vi "Event-Driven State Machine - Handle Error Locally.vi"() -> ()   [LabVIEW 2020]
uses:
  support/States.ctl
  support/State Machine Data.ctl
  <vilib>/DAQmx/read.llb/DAQmx Read (Analog 2D DBL NChan NSamp).vi
  <vilib>/DAQmx/write.llb/DAQmx Write (Analog DBL 1Chan 1Samp).vi
  <vilib>/DAQmx/create/channels.llb/DAQmx Create Channel (AI-Voltage-Basic).vi
  <vilib>/DAQmx/configure/timing.llb/DAQmx Timing (Sample Clock).vi
  <vilib>/DAQmx/miscellaneous.llb/DAQmx Fill In Error Info.vi
  <vilib>/Utility/file.llb/Write Delimited Spreadsheet (DBL).vi
  <vilib>/DAQmx/create/channels.llb/DAQmx Create Channel (AO-Voltage-Basic).vi
panel:
  in  "AO Voltage Channel":tag="PCI-6221/ao1"
  in  "Generate Stimulus":bool
  out "Threshold exceeded?":bool
  in  "Acquire":bool
  in  "Samples per channel":i32=100
  in  "Sample Rate (Hz)":dbl=1000.0
  in  "AI Voltage Channel":tag="PCI-6221/ai0, PCI-6221/ai2:3"
  in  "Threshold (rms)":dbl=1.0
  in  "Clear":bool
  in  "Exit":bool
  out "Graph":dbl[][](graph)
  # "Analysis"
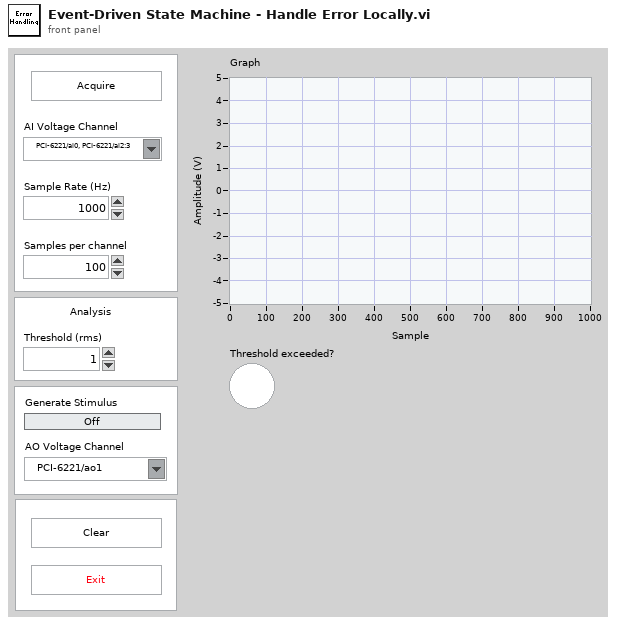
[diagram p1: front panel]
types:
  T1 = typedef "State Machine Data.ctl" = cluster{"Acquisition Data":dbl[][], "Stimulus Value":bool}
  T2 = typedef "States.ctl" = enum16{"Initialize", "Wait for Event", "Acquire", "Analyze", "Log", "Clear", "Update Graph", "Update Stumulus", "Exit"}
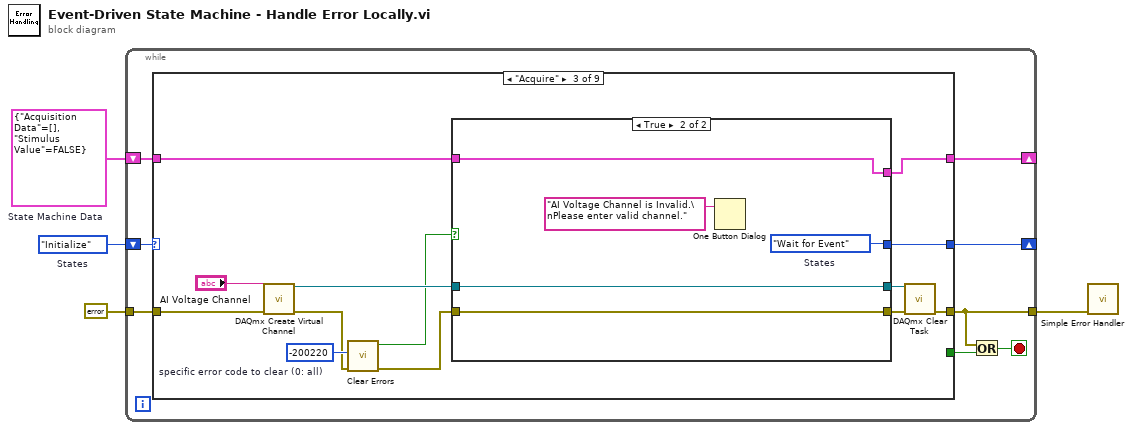
[diagram p0: block diagram]
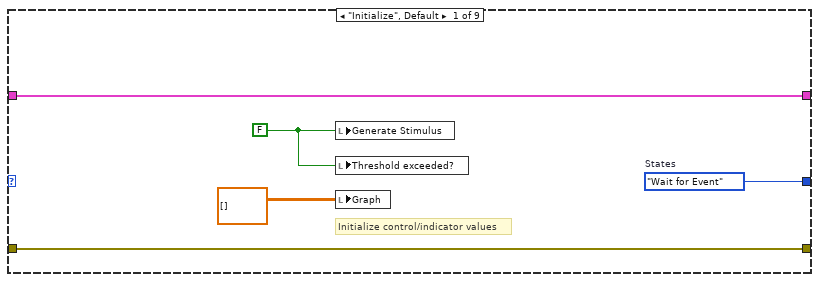
[diagram p2: hidden frame]
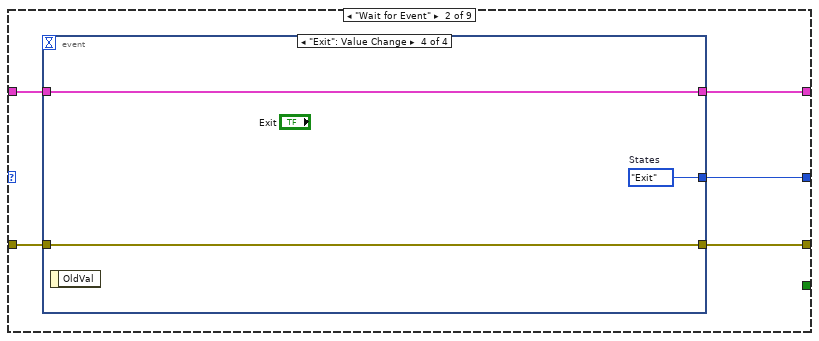
[diagram p3: hidden frame]
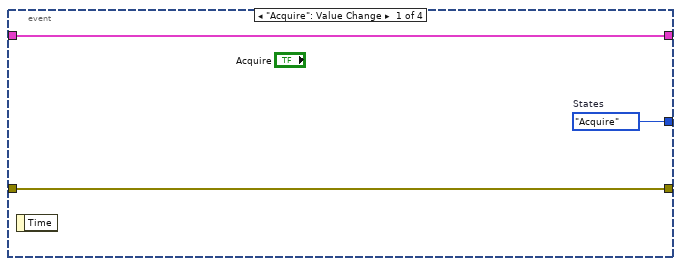
[diagram p4: hidden frame]
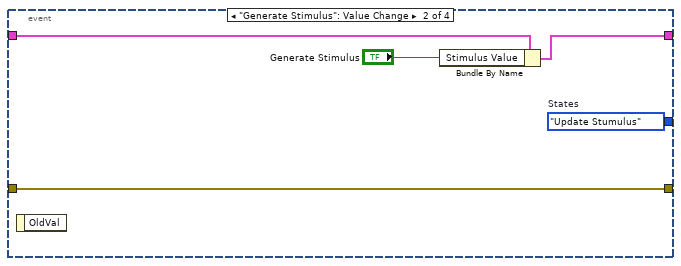
[diagram p5: hidden frame]
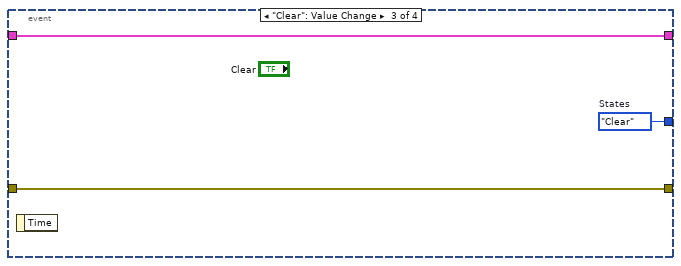
[diagram p6: hidden frame]
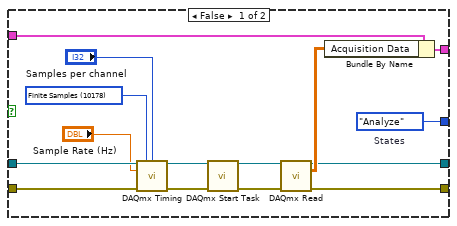
[diagram p7: hidden frame]
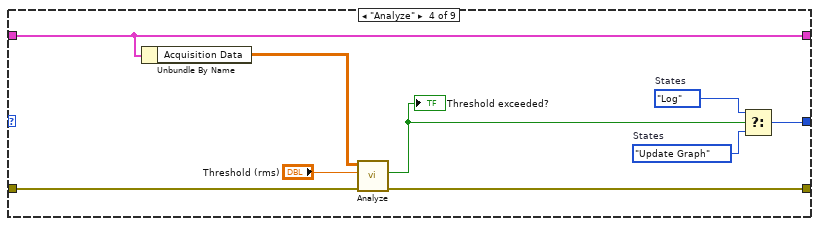
[diagram p8: hidden frame]
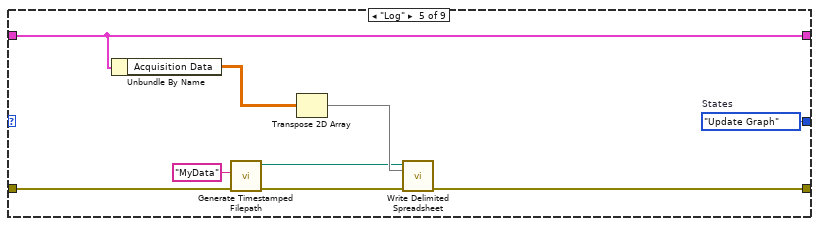
[diagram p9: hidden frame]
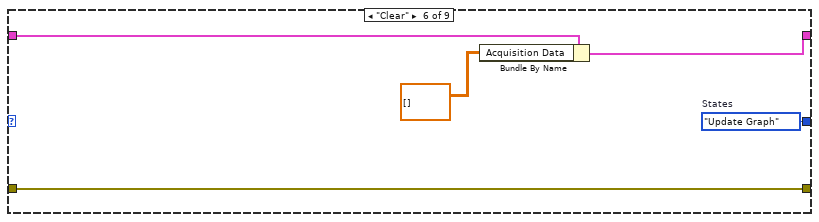
[diagram p10: hidden frame]
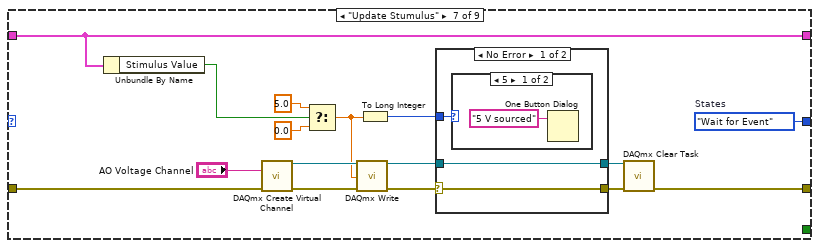
[diagram p11: hidden frame]
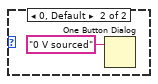
[diagram p12: hidden frame]
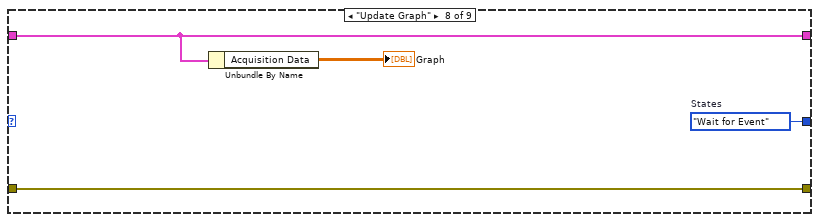
[diagram p14: hidden frame]
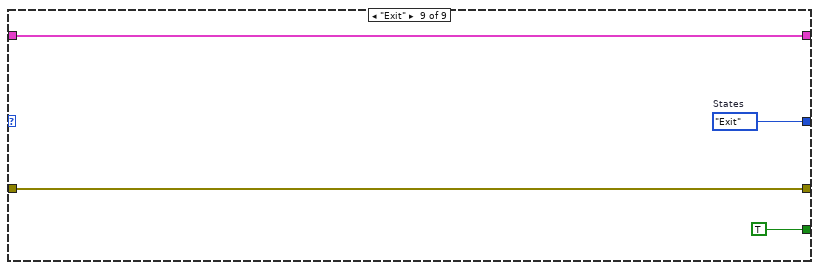
[diagram p15: hidden frame]
diagram:
  w4 = T1 {"Acquisition Data"=[], "Stimulus Value"=FALSE}  # State Machine Data
  w3 = States."Initialize"  # States
  n1 = while {
    tunnel: errorcluster {"status"=FALSE, "code"=0, "source"=""} ("error constant") -> [w11]
    tunnel: [w7] -> w1
    shift-right: [w9] -> _
    shift-left: w4 -> [w10]
    shift-right: [w8] -> _
    shift-left: w3 -> [w12]
    stop <- w6 stop-if-true
    n2 = case shown="\"Acquire\"" w12 {
      tunnel: w11 -> [w17 w20 w49 w77 w86 w92 w98 w118 w122]
      tunnel: [w17 w19 w47 w76 w80 w92 w93 w118 w122] -> w7
      tunnel: [w16 w21 w45 w78 w87 w90 w108 w119 w123] -> w9
      tunnel: w10 -> [w16 w22 w46 w78 w87 w91 w108 w119 w123]
      tunnel: [w15 w18 w41 w72 w79 w88 w99 w117 w120] -> w8
      tunnel: [_ _ _ _ _ _ _ _ TRUE] -> w5
      frame "Initialize", Default {
        w14 = FALSE
        w15 = States."Wait for Event"  # States
        # "Initialize control/indicator values"
        n3 = local write "Generate Stimulus"(w14) -> ()
        n4 = local write "Threshold exceeded?"(w14) -> ()
        n5 = local write "Graph"(dbl[][] []) -> ()
      }
      frame "Wait for Event" {
        n6 = event shown="[3] \"Exit\": Value Change" {
          selector: _ -> [_ _ _ _]
          dyn-events: _ -> [_ _ _ _]
          timeout: _ -> [_ _ _ _]
          tunnel: w22 -> [w25 w30 w33 w35]
          tunnel: [w25 w29 w33 w35] -> w21
          tunnel: w20 -> [w24 w26 w32 w36]
          tunnel: [w24 w26 w32 w36] -> w19
          tunnel: [w23 w27 w31 w34] -> w18
          event "Acquire": Value Change {
            w23 = States."Acquire"  # States
            n7 = event-data() -> ()  [unwired: 1 in, 1 out]
          }
          event "Generate Stimulus": Value Change {
            w27 = States."Update Stumulus"  # States
            n8 = event-data() -> ()  [unwired: 1 in, 1 out]
            n9 = Bundle By Name(cluster=w30, "Stimulus Value"="Generate Stimulus") -> (w29:T1)
          }
          event "Clear": Value Change {
            w31 = States."Clear"  # States
            n10 = event-data() -> ()  [unwired: 1 in, 1 out]
          }
          event "Exit": Value Change {
            w34 = States."Exit"  # States
            n11 = event-data() -> ()  [unwired: 1 in, 1 out]
          }
        }
      }
      frame "Acquire" {
        w40 = -200220  # specific error code to clear (0: all)
        n12 = call-poly <vilib>:"DAQmx Create Virtual Channel.vi"("physical channels"="AI Voltage Channel", "error in"=w49) -> ("task out"=w43:refnum<k21>, "error out"=w39:errorcluster)  [unwired: 12 in]
        n13 = call <vilib>:"Clear Errors.vi"("error in (no error)"=w39, "specific error code to clear (0: all)"=w40) -> ("error out"=w38:errorcluster, "specific error cleared?"=w37:bool)  [unwired: 4 in]
        n14 = case shown="True" w37 {
          tunnel: w38 -> [w64 w67]
          tunnel: [w61 w67] -> w48
          tunnel: w46 -> [w60 w69]
          tunnel: [w59 w69] -> w45
          tunnel: w43 -> [w55 w68]
          tunnel: [w52 w68] -> w42
          tunnel: [w50 w66] -> w41
          frame False {
            w50 = States."Analyze"  # States
            w58 = 10178 items=["Finite Samples"=10178, "Continuous Samples"=10123, "Hardware Timed Single Point"=12522] ("sample mode")
            n15 = call-poly <vilib>:"DAQmx Timing.vi"("task/channels in"=w55, "sample mode"=w58, "samples per channel"="Samples per channel", "rate"="Sample Rate (Hz)", "error in"=w64) -> ("task out"=w54:refnum<k21>, "error out"=w63:errorcluster)  [unwired: 9 in]
            n16 = call <vilib>:"DAQmx Start Task.vi"("task/channels in"=w54, "error in"=w63) -> ("task out"=w53:refnum<k21>, "error out"=w62:errorcluster)  [unwired: 12 in]
            n17 = call-poly <vilib>:"DAQmx Read.vi"("task/channels in"=w53, "error in"=w62) -> ("task out"=w52:refnum<k21>, "data"=w56:dbl[][], "error out"=w61:errorcluster)  [unwired: 11 in]
            n18 = Bundle By Name(cluster=w60, "Acquisition Data"=w56) -> (w59:T1)
          }
          frame True {
            w66 = States."Wait for Event"  # States
            n19 = One Button Dialog(message="AI Voltage Channel is Invalid.\nPlease enter valid channel.") -> ()  [unwired: 1 in, 1 out]
          }
        }
        n20 = call <vilib>:"DAQmx Clear Task.vi"("task in"=w42, "error in"=w48) -> ("error out"=w47:errorcluster)  [unwired: 13 in]
      }
      frame "Analyze" {
        w73 = States."Update Graph"  # States
        w74 = States."Log"  # States
        n21 = Unbundle By Name(w78) -> ("Acquisition Data"=w75:dbl[][])
        n22 = call "Analyze.vi"("Error In"=w77, "Treshold (rms)"="Threshold (rms)", "N-Channel Data (2D DBL)"=w75) -> ("Error Out"=w76:errorcluster, "Threshold exceeded?"=w70:bool)  [unwired: 5 in, 2 out]
        "Threshold exceeded?" <- w70
        n23 = Select(t=w74, s=w70, f=w73) -> (s? t:f=w72:T2)
      }
      frame "Log" {
        w79 = States."Update Graph"  # States
        n24 = Unbundle By Name(w87) -> ("Acquisition Data"=w84:dbl[][])
        n25 = call "Generate Timestamped Filepath.vi"("Error In"=w86, "appended filename"="MyData") -> ("Error Out"=w81:errorcluster, "timestamped relative filepath"=w82:path)  [unwired: 8 in]
        n26 = Transpose 2D Array(2D array=w84) -> (transposed array=w83:dbl[][])
        n27 = call-poly <vilib>:"Write Delimited Spreadsheet.vi"("file path (dialog if empty)"=w82, "2D data"=w83, "error in (no error)"=w81) -> ("error out"=w80:errorcluster)  [unwired: 11 in, 1 out]
      }
      frame "Clear" {
        w88 = States."Update Graph"  # States
        n28 = Bundle By Name(cluster=w91, "Acquisition Data"=dbl[][] []) -> (w90:T1)
      }
      frame "Update Stumulus" {
        w99 = States."Wait for Event"  # States
        n29 = Unbundle By Name(w108) -> ("Stimulus Value"=w100:bool)
        n30 = call-poly <vilib>:"DAQmx Create Virtual Channel.vi"("physical channels"="AO Voltage Channel", "error in"=w98) -> ("task out"=w105:refnum<k21>, "error out"=w104:errorcluster)  [unwired: 12 in]
        n31 = Select(t=5.0, s=w100, f=0.0) -> (s? t:f=w102:dbl)
        n32 = call-poly <vilib>:"DAQmx Write.vi"("task/channels in"=w105, "data"=w102, "error in"=w104) -> ("task out"=w95:refnum<k21>, "error out"=w96:errorcluster)  [unwired: 10 in, 1 out]
        n33 = To Long Integer(number=w102) -> (32bit integer=w101:i32)
        n34 = case shown="No Error" w96 {
          selector: w96 -> [w109 w115]
          tunnel: w101 -> [w111 _]
          tunnel: [w109 w115] -> w97
          tunnel: w95 -> [w110 w114]
          tunnel: [w110 w114] -> w94
          frame No Error {
            n35 = case shown="5" w111 {
              frame 5 {
                n36 = One Button Dialog(message="5 V sourced") -> ()  [unwired: 1 in, 1 out]
              }
              frame 0, Default {
                n37 = One Button Dialog(message="0 V sourced") -> ()  [unwired: 1 in, 1 out]
              }
            }
          }
          frame Error {
          }
        }
        n38 = call <vilib>:"DAQmx Clear Task.vi"("task in"=w94, "error in"=w97) -> ("error out"=w93:errorcluster)  [unwired: 13 in]
      }
      frame "Update Graph" {
        w117 = States."Wait for Event"  # States
        n39 = Unbundle By Name(w119) -> ("Acquisition Data"=→"Graph":dbl[][])
      }
      frame "Exit" {
        w120 = States."Exit"  # States
      }
    }
    n40 = Or(x=w7, y=w5) -> (x .or. y?=w6:bool)
  }
  n41 = call <vilib>:"Simple Error Handler.vi"("error in (no error)"=w1) -> ()  [unwired: 4 in, 5 out]
